vi "RPM Conversion.vi"(11 "RPM":dbl) -> (3 "RPM Out":dbl)   [LabVIEW 2015]
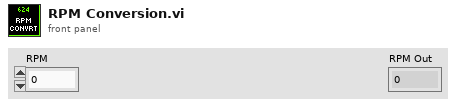
[diagram p1: front panel]
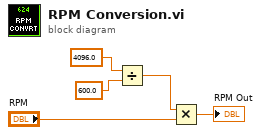
[diagram p0: block diagram]
diagram:
  n1 = Divide(x=4096.0, y=600.0) -> (x/y=w3:dbl)
  n2 = Multiply(x=w3, y="RPM") -> (x*y=→"RPM Out":dbl)
